vi "Wiimote Set LEDs.vi"(8 "error in":errorcluster, 10 "Wiimote LEDs":T1, 11 "hWiimoteHandle in":u32 format="%08x") -> (0 "error out":errorcluster, 3 "hWiimoteHandle out":u32 format="%08x")   [LabVIEW 2010]
uses:
  Wiimote LEDs.ctl
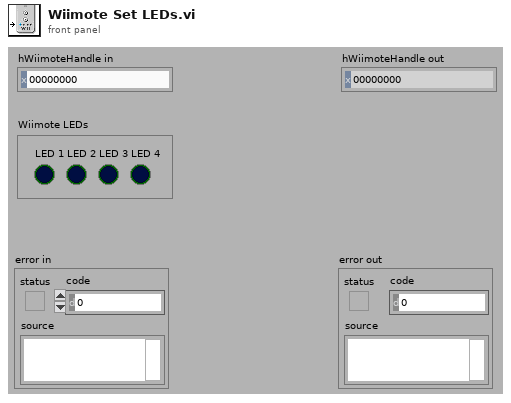
[diagram p1: front panel]
types:
  T1 = typedef "Wiimote LEDs.ctl" = cluster{"LED 1":bool, "LED 2":bool, "LED 3":bool, "LED 4":bool}
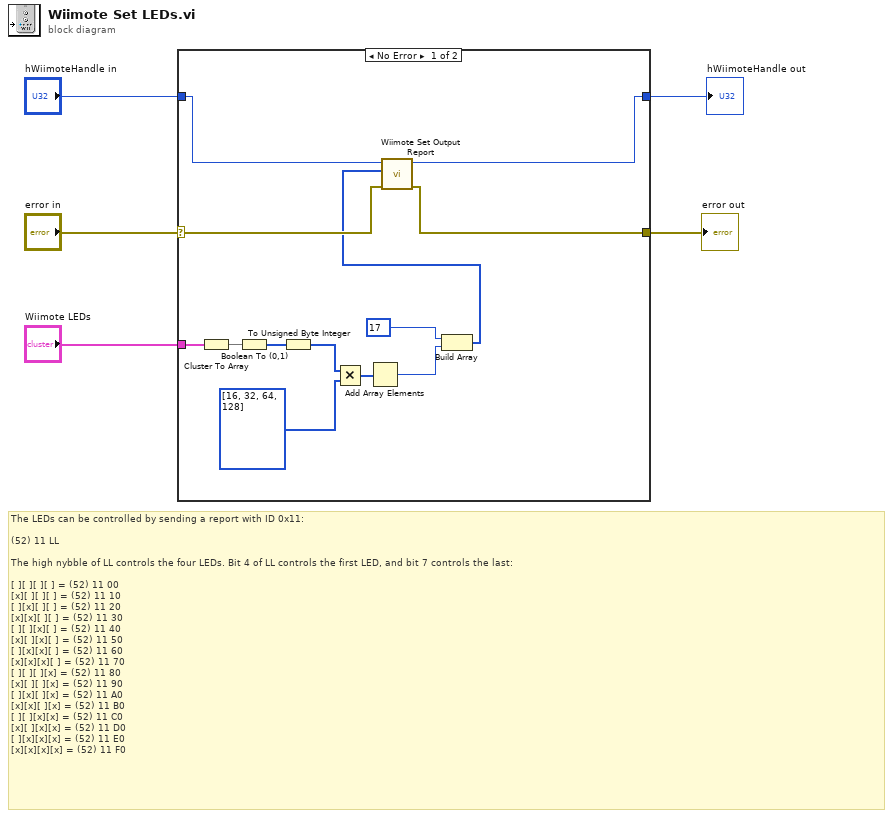
[diagram p0: block diagram]
diagram:
  # "The LEDs can be controlled by sending a report with ID 0x11:\n\n(52) 11 LL\n\nThe high nybble of LL controls the four LEDs. Bit 4 of LL controls the first LED, and bit 7 controls the last:\n\n[ ][ ][ ][ ] = (52) 11 00\n[x][ ][ ][ ] = (52) 11 10\n[ ][x][ ][ ] = (52) 11 20\n[x][x][ ][ ] = (52) 11 30\n[ ][ ][x][ ] = (52) 11 40\n[x][ ][x][ ] = (52) 11 50\n[ ][x][x][ ] = (52) 11 60\n[x][x][x][ ] = (52) 11 70\n[ ][ ][ ][x] = (52) 11 80\n[x][ ][ ][x] = (52) 11 90\n[ ][x][ ][x] = (52) 11 A0\n[x][x][ ][x] = (52) 11 B0\n[ ][ ][x][x] = (52) 11 C0\n[x][ ][x][x] = (52) 11 D0\n[ ][x][x][x] = (52) 11 E0\n[x][x][x][x] = (52) 11 F0"
  n1 = case shown="No Error" "error in" {
    selector: "error in" -> [w8 w20]
    tunnel: [w7 w20] -> w4
    tunnel: "hWiimoteHandle in" -> [w10 w19]
    tunnel: [w9 w19] -> w2
    tunnel: "Wiimote LEDs" -> [w18 _]
    frame No Error {
      n2 = Cluster To Array(cluster=w18) -> (array=w17:bool[])
      n3 = Boolean To (0,1)(Boolean=w17) -> (0, 1=w16:i16[])
      n4 = To Unsigned Byte Integer(number=w16) -> (unsigned 8bit integer=w14:u8[])
      n5 = Multiply(x=w14, y=u8[] [16, 32, 64, 128]) -> (x*y=w13:u8[])
      n6 = Add Array Elements(numeric array=w13) -> (sum=w11:u8)
      n7 = Build Array(u8 17, w11) -> (w6:u8[])
      n8 = call "Wiimote Set Output Report.vi"("error in"=w8, "pReportBuffer in"=w6, "hWiimoteHandle in"=w10) -> ("error out"=w7:errorcluster, "hWiimoteHandle out"=w9:u32)  [unwired: 7 in]
    }
    frame Error {
    }
  }
  "error out" <- w4
  "hWiimoteHandle out" <- w2
